vi "Step of KeFo params.vi"(7 "Step of KeepForce params":T1, 8 "error in (no error)":errorcluster, 10 "Step NO":u8=1 min=1 max=50 step=1, 11 "Profile NO":u8=1 min=1 max=50 step=1) -> (0 "error out":errorcluster, 2 "wchitch params":string, 3 "params array out":string[](array[string]))   [LabVIEW 2019, in "STAV lib.lvlib"]
uses:
  STAV lib.lvlib
  Step of KeFo params.ctl
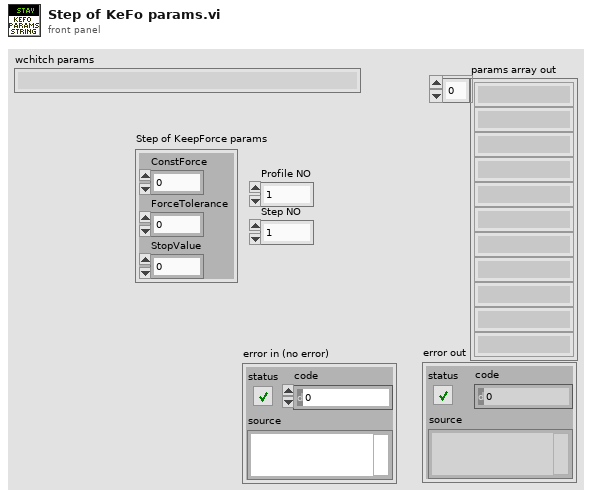
[diagram p1: front panel]
types:
  T1 = typedef "STAV lib.lvlib/Step of KeFo params.ctl" = cluster{"ConstForce":dbl, "ForceTolerance":dbl, "StopValue":dbl}
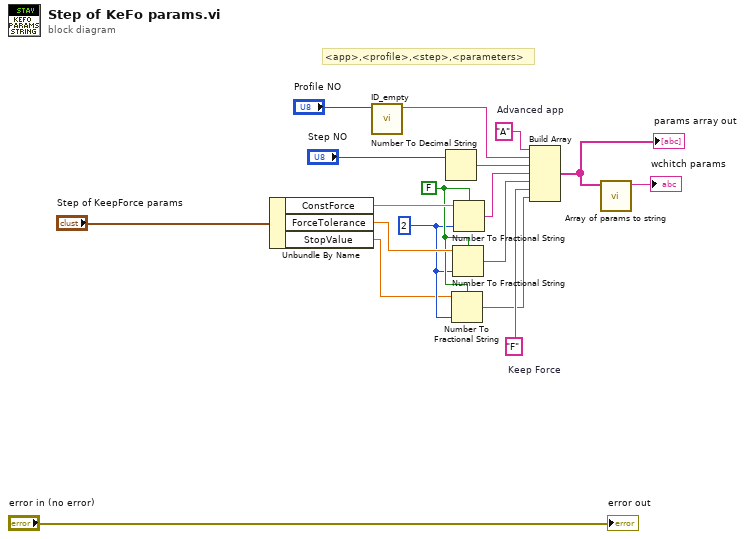
[diagram p0: block diagram]
diagram:
  w5 = "F"  # Keep Force
  w3 = i16 2 ("precision (6)")
  w4 = FALSE ("use system decimal point (T)")
  w18 = "A"  # Advanced app
  # "<app>,<profile>,<step>,<parameters>"
  n1 = Unbundle By Name("Step of KeepForce params") -> ("ConstForce"=w8:dbl, "ForceTolerance"=w6:dbl, "StopValue"=w2:dbl)
  n2 = call "ID_empty.vi"("Profile NO"="Profile NO") -> ("Profile NO out"=w15:string)  [unwired: 9 in, 1 out]
  n3 = Number To Decimal String(number="Step NO") -> (decimal integer string=w11:string)  [unwired: 1 in]
  n4 = Number To Fractional String(use system decimal point (T)=w4, number=w2, precision (6)=w3) -> (F-format string=w1:string)  [unwired: 1 in]
  n5 = Number To Fractional String(use system decimal point (T)=w4, number=w6, precision (6)=w3) -> (F-format string=w7:string)  [unwired: 1 in]
  n6 = Number To Fractional String(use system decimal point (T)=w4, number=w8, precision (6)=w3) -> (F-format string=w10:string)  [unwired: 1 in]
  n7 = Build Array(w18, w15, w11, w10, w7, w5, w1) -> (w14:string[])
  "params array out" <- w14
  n8 = call "Array of params to string.vi"("Array"=w14) -> ("String"=→"wchitch params":string)  [unwired: 10 in]
  "error out" <- "error in (no error)"
